vi "Process.vi"(11 "Actor":refnum<class "Debugger.lvclass">) -> ()   [LabVIEW 2021, in "Debugger.lvclass"]
uses:
  Debugger.lvclass
  Debugger.lvclass/Debugger.ctl
  Base Actor/Actor/Front Panel State.ctl
  Base Actor/Actor/Actor.lvclass
  Messaging/Message/Message.lvclass
  Application Specific/Actors/Error Handler/API/Error Handler Actor API.lvclass
  Utility/Utility.lvlib
  Debug Tools/Actor Ref Cache/Actor Ref Cache Action.ctl
  Action.ctl
panel:
  in  "Update":bool
  in  "Up":bool
  in  "Left":bool
  in  "Right":bool
  in  "Down":bool
  in  "Abort All":bool
  in  "Action":T1=enum."Open BD"
  out "error out":errorcluster
  in  "Actors":i32(listbox)=-1
  in  "Show Metronomes":bool
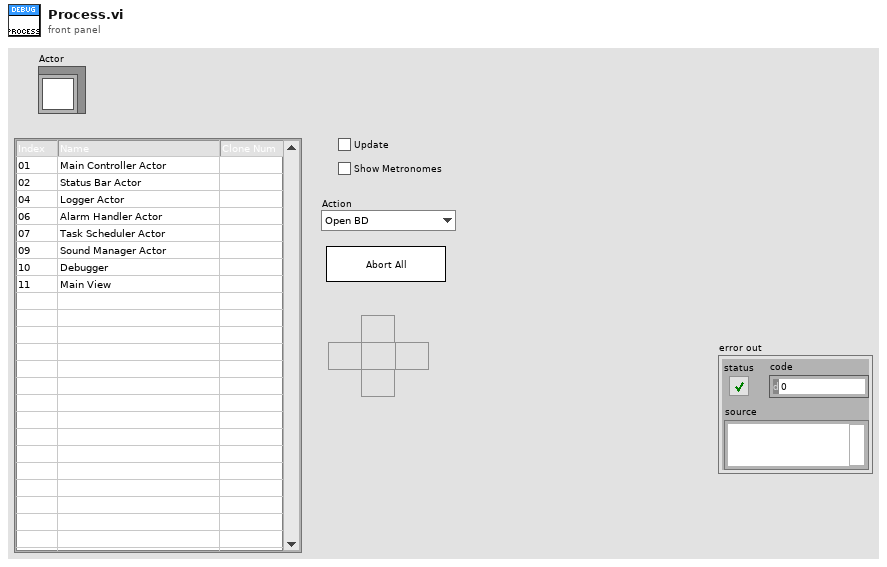
[diagram p1: front panel]
types:
  T1 = typedef "Debugger.lvclass/Action.ctl" = enum16{"Open FP", "Close FP", "Open BD", "Close BD", "Abort", "Enable Toolbar", "Move FP Up", "Move FP Down", "Move FP Left", "Move FP Right"}
  T2 = typedef "Actor.lvclass/Front Panel State.ctl" = enum32{"Invalid", "Standard", "Closed", "Hidden", "Minimized", "Maximized"}
  T3 = typedef "Actor Ref Cache Action.ctl" = enum16{"Clear", "Add Ref", "Remove Ref", "Get All Refs"}
  T4 = typedef "LVPoint32TypeDef.ctl" = cluster{"Horizontal":i32, "Vertical":i32}
  T5 = enum32{"invalid app kind", "Development System", "Run Time System", "Student Edition", "Embedded LabVIEW", "Evaluation", "Custom"}
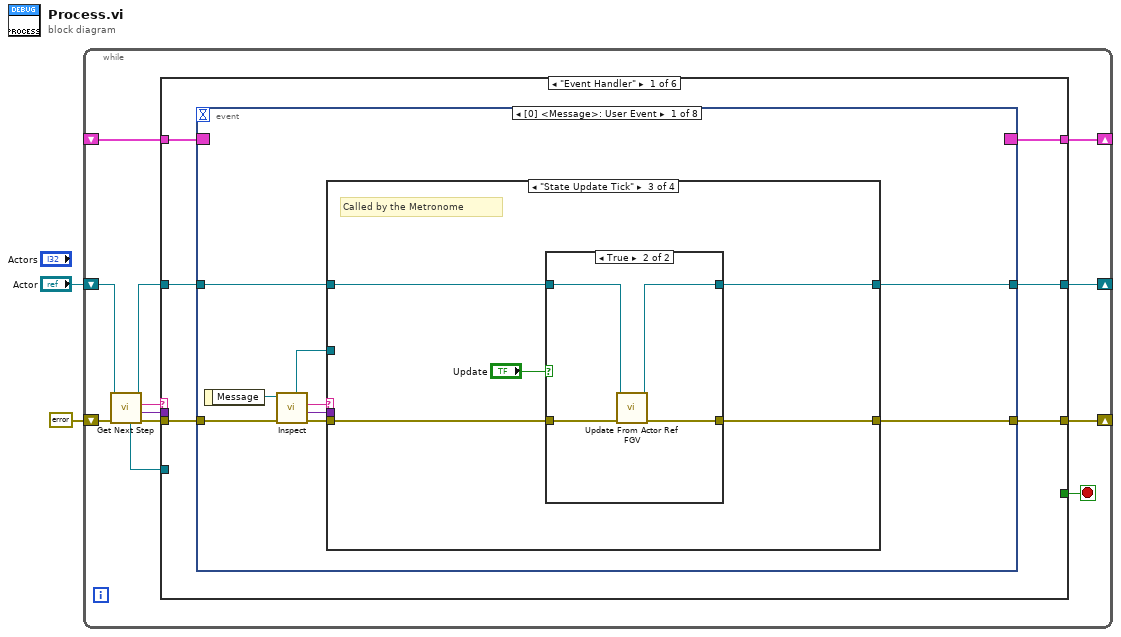
[diagram p0: block diagram]
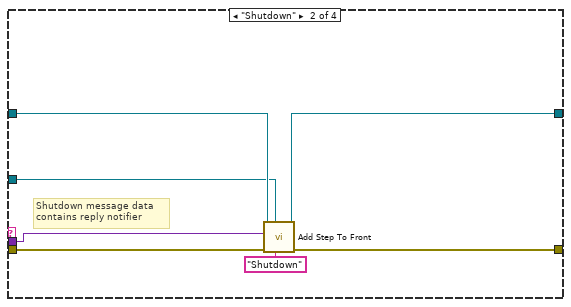
[diagram p3: hidden frame]
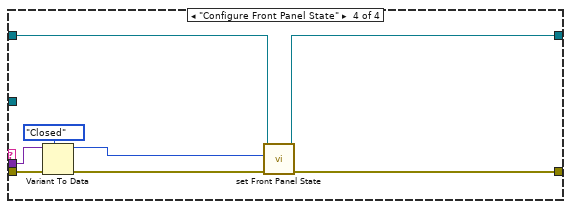
[diagram p5: hidden frame]
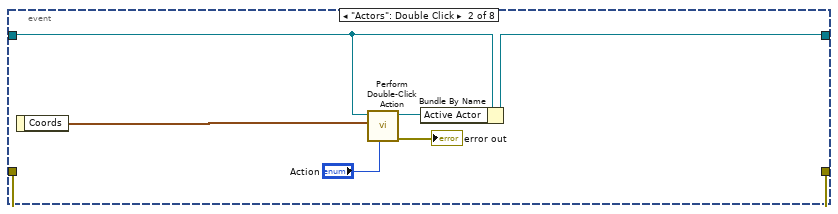
[diagram p6: hidden frame]
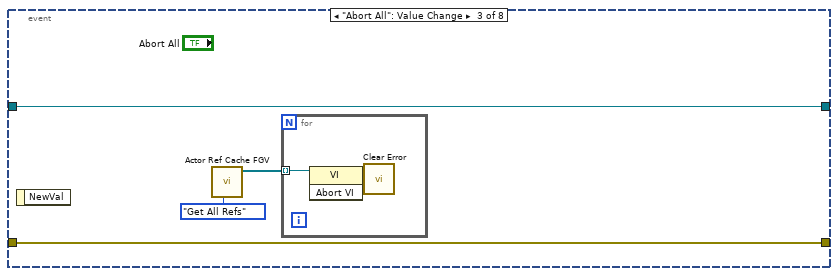
[diagram p7: hidden frame]
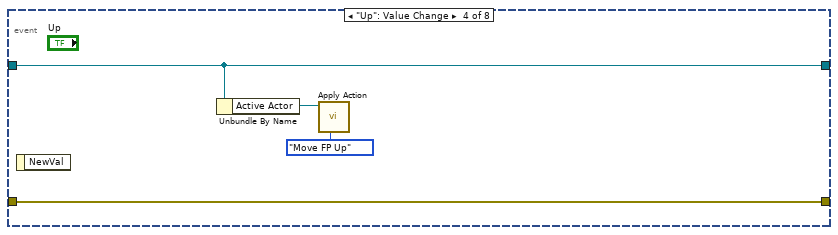
[diagram p8: hidden frame]
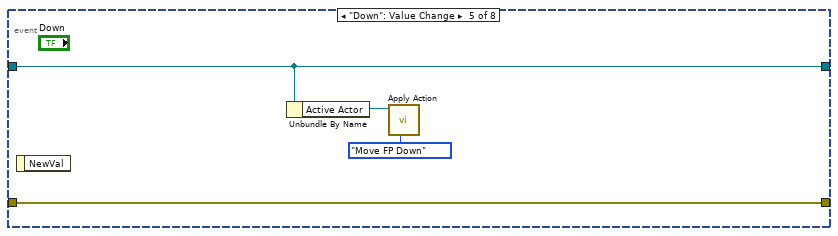
[diagram p9: hidden frame]
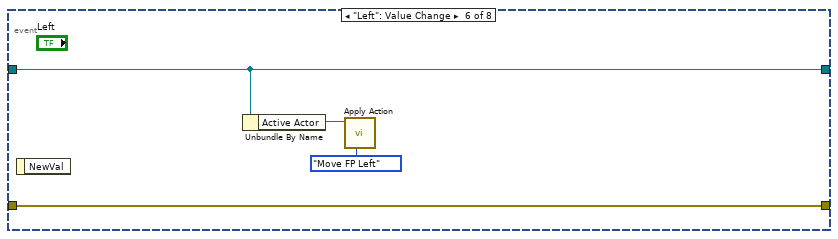
[diagram p10: hidden frame]
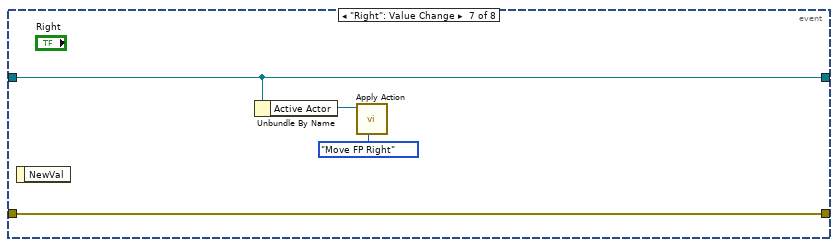
[diagram p11: hidden frame]
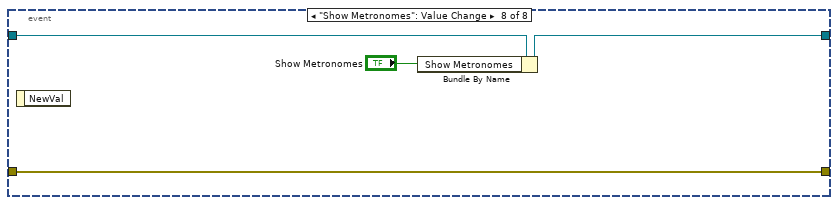
[diagram p12: hidden frame]
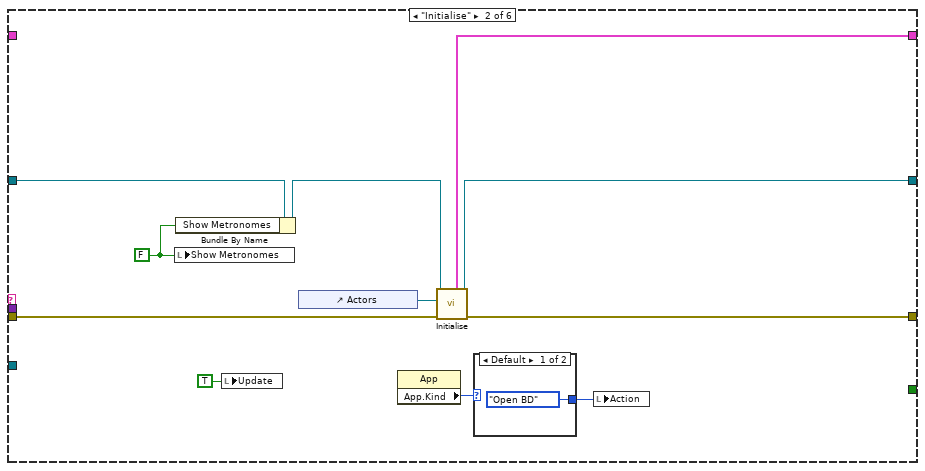
[diagram p13: hidden frame]
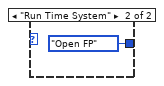
[diagram p14: hidden frame]
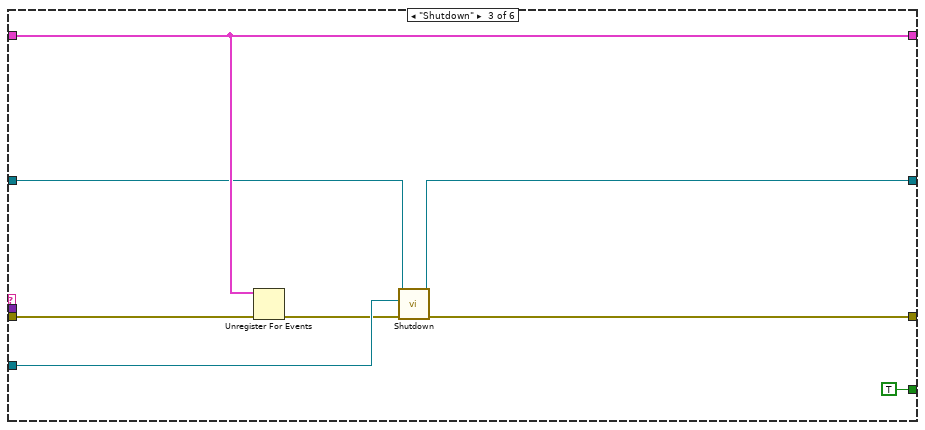
[diagram p15: hidden frame]
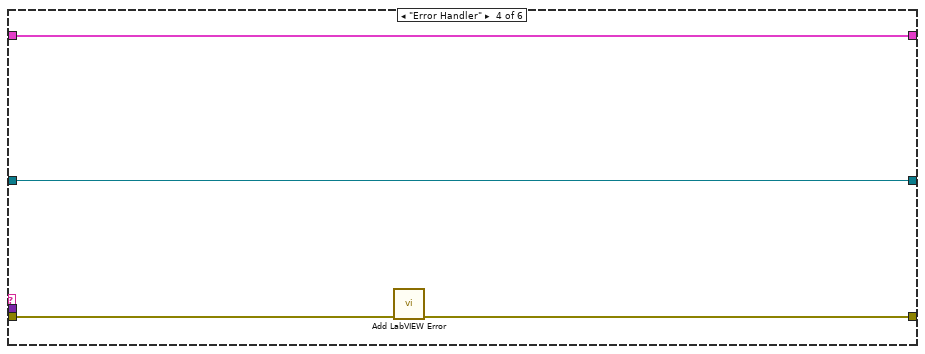
[diagram p16: hidden frame]
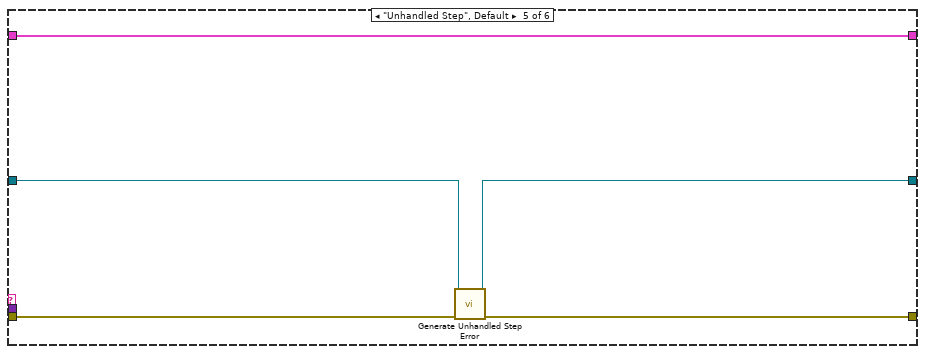
[diagram p17: hidden frame]
diagram:
  n1 = while {
    shift-right: [w5] -> _
    shift-left: "Actor" -> [w13]
    shift-right: [w10] -> _
    shift-left: _ -> [w9]
    shift-right: [w4] -> _
    shift-left: errorcluster {"status"=FALSE, "code"=0, "source"=""} ("error constant") -> [w7]
    stop <- w14 stop-if-true
    n2 = call-dynamic "Get Next Step.vi"("error in (no error)"=w7, "Actor in"=w13) -> ("error out"=w8:errorcluster, "Parameter"=w11:variant, "Step"=w6:string, "Actor out"=w12:refnum<class "Debugger.lvclass">, "Reply Channel"=w3:refnum<notifier>)  [unwired: 5 in]
    n3 = case shown="\"Event Handler\"" w6 {
      tunnel: [_ _ TRUE _ _ _] -> w14
      tunnel: w12 -> [w20 w93 w109 w112 w119 w122]
      tunnel: [w19 w98 w108 w112 w118 w122] -> w5
      tunnel: w11 -> [_ _ _ _ _ _]
      tunnel: [w17 w101 w110 w115 w120 w123] -> w10
      tunnel: w9 -> [w18 _ w110 w115 w120 w123]
      tunnel: w8 -> [w16 w99 w106 w114 w117 w121]
      tunnel: [w15 w100 w104 w113 w116 w121] -> w4
      tunnel: w3 -> [_ _ w107 _ _ _]
      frame "Event Handler" {
        n4 = event shown="[0] <Message>: User Event" {
          selector: w18 -> [_ _ _ _ _ _ _ _]
          dyn-events: [_ _ _ _ _ _ _ _] -> w17
          timeout: _ -> [_ _ _ _ _ _ _ _]
          tunnel: w20 -> [w29 w61 w68 w71 w75 w81 w83 w89]
          tunnel: [w28 w62 w68 w71 w75 w81 w83 w88] -> w19
          tunnel: w16 -> [w26 w64 w67 w74 w78 w82 w86 w90]
          tunnel: [w27 w64 w67 w74 w78 w82 w86 w90] -> w15
          event User Event {
            n5 = event-data() -> ("Message"=w25:refnum<class "Message.lvclass">)  [unwired: 1 in]
            n6 = call "Inspect.vi"("error in (no error)"=w26, "Message in"=w25) -> ("error out"=w22:errorcluster, "Data"=w23:variant, "Name"=w24:string, "Reply Channel"=w21:refnum<notifier>)  [unwired: 5 in, 1 out]
            n7 = case shown="\"State Update Tick\"" w24 {
              tunnel: w29 -> [w31 w38 w43 w57]
              tunnel: [w31 w37 w42 w56] -> w28
              tunnel: w22 -> [w30 w35 w41 w53]
              tunnel: [w30 w34 w40 w55] -> w27
              tunnel: w23 -> [_ w33 _ w54]
              tunnel: w21 -> [_ w32 _ _]
              frame Default {
              }
              frame "Shutdown" {
                # "Shutdown message data contains reply notifier"
                n8 = call-dynamic "Add Step To Front.vi"("Step Name"="Shutdown", "Reply Channel"=w32, "error in (no error)"=w35, "Parameter"=w33, "Actor in"=w38) -> ("error out"=w34:errorcluster, "Actor out"=w37:refnum<class "Debugger.lvclass">)  [unwired: 5 in]
              }
              frame "State Update Tick" {
                # "Called by the Metronome"
                n9 = case shown="True" "Update" {
                  tunnel: w43 -> [w45 w47]
                  tunnel: [w45 w46] -> w42
                  tunnel: w41 -> [w44 w49]
                  tunnel: [w44 w48] -> w40
                  frame False {
                  }
                  frame True {
                    n10 = call "Update From Actor Ref FGV.vi"("error in (no error)"=w49, "Debugger in"=w47) -> ("error out"=w48:errorcluster, "Debugger out"=w46:refnum<class "Debugger.lvclass">)  [unwired: 8 in]
                  }
                }
              }
              frame "Configure Front Panel State" {
                n11 = Variant To Data(error in=w53, type=Front_Panel_State."Closed" ("Front Panel State"), Variant=w54) -> (data=w50:T2, error out=w52:errorcluster)
                n12 = call-dynamic "set Front Panel State.vi"("error in (no error)"=w52, "Front Panel State"=w50, "Actor in"=w57) -> ("error out"=w55:errorcluster, "Actor out"=w56:refnum<class "Debugger.lvclass">)  [unwired: 7 in]
              }
            }
          }
          event "Actors": Double Click {
            n13 = event-data() -> ("Coords"=w60:T4)  [unwired: 1 in]
            n14 = call "Perform Double-Click Action.vi"("Action"="Action", "Coords"=w60, "Debugger"=w61) -> ("error out"=→"error out":errorcluster, "Selected Actor"=w58:refnum<vi>)  [unwired: 7 in]
            n15 = Bundle By Name(cluster=w61, "Active Actor"=w58) -> (w62:refnum<class "Debugger.lvclass">)
          }
          event "Abort All": Value Change {
            n16 = event-data() -> ()  [unwired: 1 in, 1 out]
            n17 = call "Actor Ref Cache FGV.vi"("Action"=Actor_Ref_Cache_Action."Get All Refs") -> ("All Refs Out"=w66:refnum<vi>[])  [unwired: 10 in]
            n18 = for {
              tunnel: w66 -> [w70] mode=indexing
              n19 = invoke class="VI" method="Abort VI"(reference=w70) -> (error out=w69:errorcluster)  [unwired: 2 in, 2 out]
              n20 = call "Clear Error.vi"("error in (no error)"=w69) -> ()  [unwired: 1 out]
            }
          }
          event "Up": Value Change {
            n21 = event-data() -> ()  [unwired: 1 in, 1 out]
            n22 = Unbundle By Name(w71) -> ("Active Actor"=w72:refnum<vi>)
            n23 = call "Apply Action.vi"("Action"=Action."Move FP Up", "VI Refnum"=w72) -> ()  [unwired: 9 in, 1 out]
          }
          event "Down": Value Change {
            n24 = event-data() -> ()  [unwired: 1 in, 1 out]
            n25 = Unbundle By Name(w75) -> ("Active Actor"=w76:refnum<vi>)
            n26 = call "Apply Action.vi"("Action"=Action."Move FP Down", "VI Refnum"=w76) -> ()  [unwired: 9 in, 1 out]
          }
          event "Left": Value Change {
            n27 = event-data() -> ()  [unwired: 1 in, 1 out]
            n28 = Unbundle By Name(w81) -> ("Active Actor"=w79:refnum<vi>)
            n29 = call "Apply Action.vi"("Action"=Action."Move FP Left", "VI Refnum"=w79) -> ()  [unwired: 9 in, 1 out]
          }
          event "Right": Value Change {
            n30 = event-data() -> ()  [unwired: 1 in, 1 out]
            n31 = Unbundle By Name(w83) -> ("Active Actor"=w84:refnum<vi>)
            n32 = call "Apply Action.vi"("Action"=Action."Move FP Right", "VI Refnum"=w84) -> ()  [unwired: 9 in, 1 out]
          }
          event "Show Metronomes": Value Change {
            n33 = event-data() -> ()  [unwired: 1 in, 1 out]
            n34 = Bundle By Name(cluster=w89, "Show Metronomes"="Show Metronomes") -> (w88:refnum<class "Debugger.lvclass">)
          }
        }
      }
      frame "Initialise" {
        w91 = FALSE ("Show Metronomes")
        n35 = local write "Show Metronomes"(w91) -> ()
        n36 = Bundle By Name(cluster=w93, "Show Metronomes"=w91) -> (w92:refnum<class "Debugger.lvclass">)
        n37 = local write "Update"(TRUE ("Update")) -> ()
        n38 = control-ref of="Actors"() -> (w97:refnum<vi>)
        n39 = property class="App"() -> ("App.Kind"=w96:T5)  [unwired: 2 in, 2 out]
        n40 = call "Initialise.vi"("error in (no error)"=w99, "Actors"=w97, "Actor in"=w92) -> ("error out"=w100:errorcluster, "Actor out"=w98:refnum<class "Debugger.lvclass">, "Observers"=w101:cluster{"Actor":refnum<event-registration>})  [unwired: 6 in]
        n41 = case shown="Default" w96 {
          tunnel: [Action."Open BD" ("Action") Action."Open FP" ("Action")] -> w95
          frame Default {
          }
          frame "Run Time System" {
          }
        }
        n42 = local write "Action"(w95) -> ()
      }
      frame "Shutdown" {
        n43 = Unregister For Events(event registration refnum=w110, error in=w106) -> (error out=w105:errorcluster)
        n44 = call-dynamic "Shutdown.vi"("error in (no error)"=w105, "Reply Channel"=w107, "Actor in"=w109) -> ("error out"=w104:errorcluster, "Actor out"=w108:refnum<class "Debugger.lvclass">)  [unwired: 7 in]
      }
      frame "Error Handler" {
        n45 = call "Add LabVIEW Error.vi"("error in (no error)"=w114) -> ("error out"=w113:errorcluster)  [unwired: 10 in]
      }
      frame "Unhandled Step", Default {
        n46 = call-dynamic "Generate Unhandled Step Error.vi"("error in (no error)"=w117, "Actor in"=w119) -> ("error out"=w116:errorcluster, "Actor out"=w118:refnum<class "Debugger.lvclass">)  [unwired: 8 in]
      }
      frame "-----------------------" {
        # "Separator"
      }
    }
  }
